vi "MGI CheckValue Directory Calculate.vi"(5 "U32 Slider Ref":refnum<vi>, 7 "CheckValue Type (Checksum)":T1, 8 "error in (no error)":errorcluster, 10 "Directories to Exclude":string[](array[string]), 11 "Path":path) -> (0 "error out":errorcluster, 1 "CheckValue U32[i]":u32[](array[numeric]) format="%.0x", 2 "Relative Path[i]":path[](array[path]), 4 "Aborted?":bool)   [LabVIEW 2020]
doc: "Output an array of all files contained in the specified directory along with a CheckValue for each file. Optional Progress Bar Input is updated if wired, otherwise a progress bar dialog with abort button is shown.\n\nAuthored by Shawn Walpole\nsupport@mooregoodideas.com\nwww.mooregoodideas.com\n\nCopyright (c) 2010, Moore Good Ideas, Inc.\n\nAll rights reserved.\n\nRedistribution and use in source and binary forms, with or without modification, are permitted provided that the following conditions are met:\n\n * Redistributions of source code must retain the above copyright notice, this list of conditions and the following disclaimer.\n * Redistributions in binary form must reproduce the above copyright notice, this list of conditions and the following disclaimer in the documentation and/or other materials provided with the distribution.\n * Neither the name of Moore Good Ideas, Inc. nor the names of its contributors may be used to endorse or promote products derived from this software without specific prior written permission.\n\nTHIS SOFTWARE IS PROVIDED BY THE COPYRIGHT HOLDERS AND CONTRIBUTORS \"AS IS\" AND ANY EXPRESS OR IMPLIED WARRANTIES, INCLUDING, BUT NOT LIMITED TO, THE IMPLIED WARRANTIES OF MERCHANTABILITY AND FITNESS FOR A PARTICULAR PURPOSE ARE DISCLAIMED. IN NO EVENT SHALL THE COPYRIGHT OWNER OR CONTRIBUTORS BE LIABLE FOR ANY DIRECT, INDIRECT, INCIDENTAL, SPECIAL, EXEMPLARY, OR CONSEQUENTIAL DAMAGES (INCLUDING, BUT NOT LIMITED TO, PROCUREMENT OF SUBSTITUTE GOODS OR SERVICES; LOSS OF USE, DATA, OR PROFITS; OR BUSINESS INTERRUPTION) HOWEVER CAUSED AND ON ANY THEORY OF LIABILITY, WHETHER IN CONTRACT, STRICT LIABILITY, OR TORT (INCLUDING NEGLIGENCE OR OTHERWISE) ARISING IN ANY WAY OUT OF THE USE OF THIS SOFTWARE, EVEN IF ADVISED OF THE POSSIBILITY OF SUCH DAMAGE."
uses:
  <userlib>/_MGI/File/Checksum/MGI CheckValue Method Enum.ctl
panel:
  out "Cur File(Rel)":path
  out "ProcessedFiles":i32
  out "TotalFiles":u32
  # "Controls used for local variables"
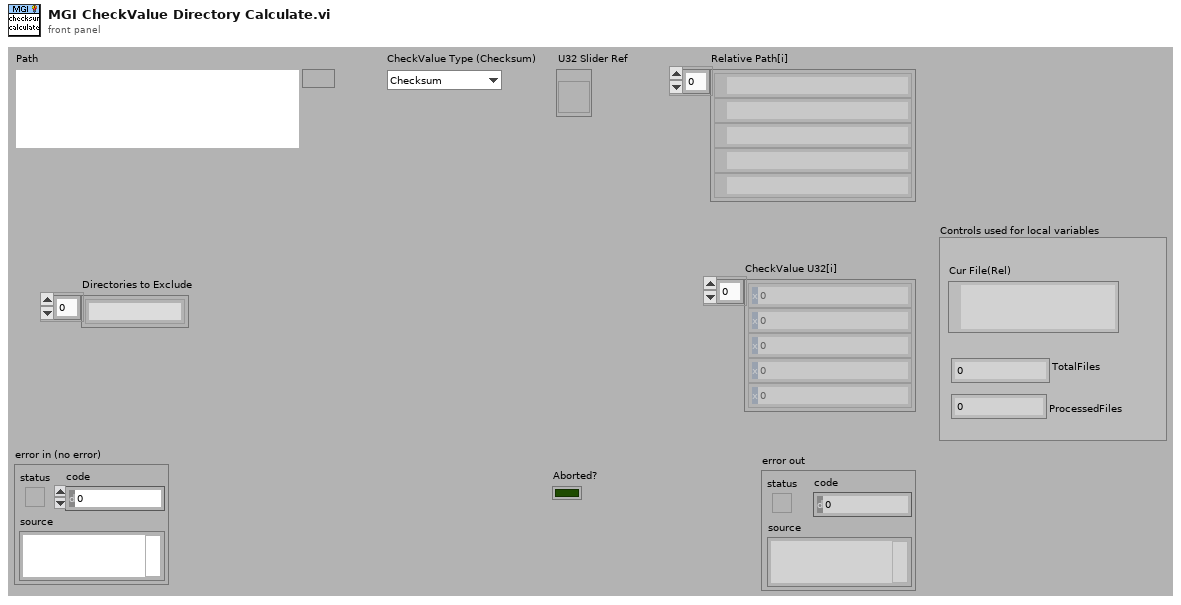
[diagram p1: front panel]
types:
  T1 = typedef "MGI CheckValue Method Enum.ctl" = enum16{"Checksum", "XOr"}
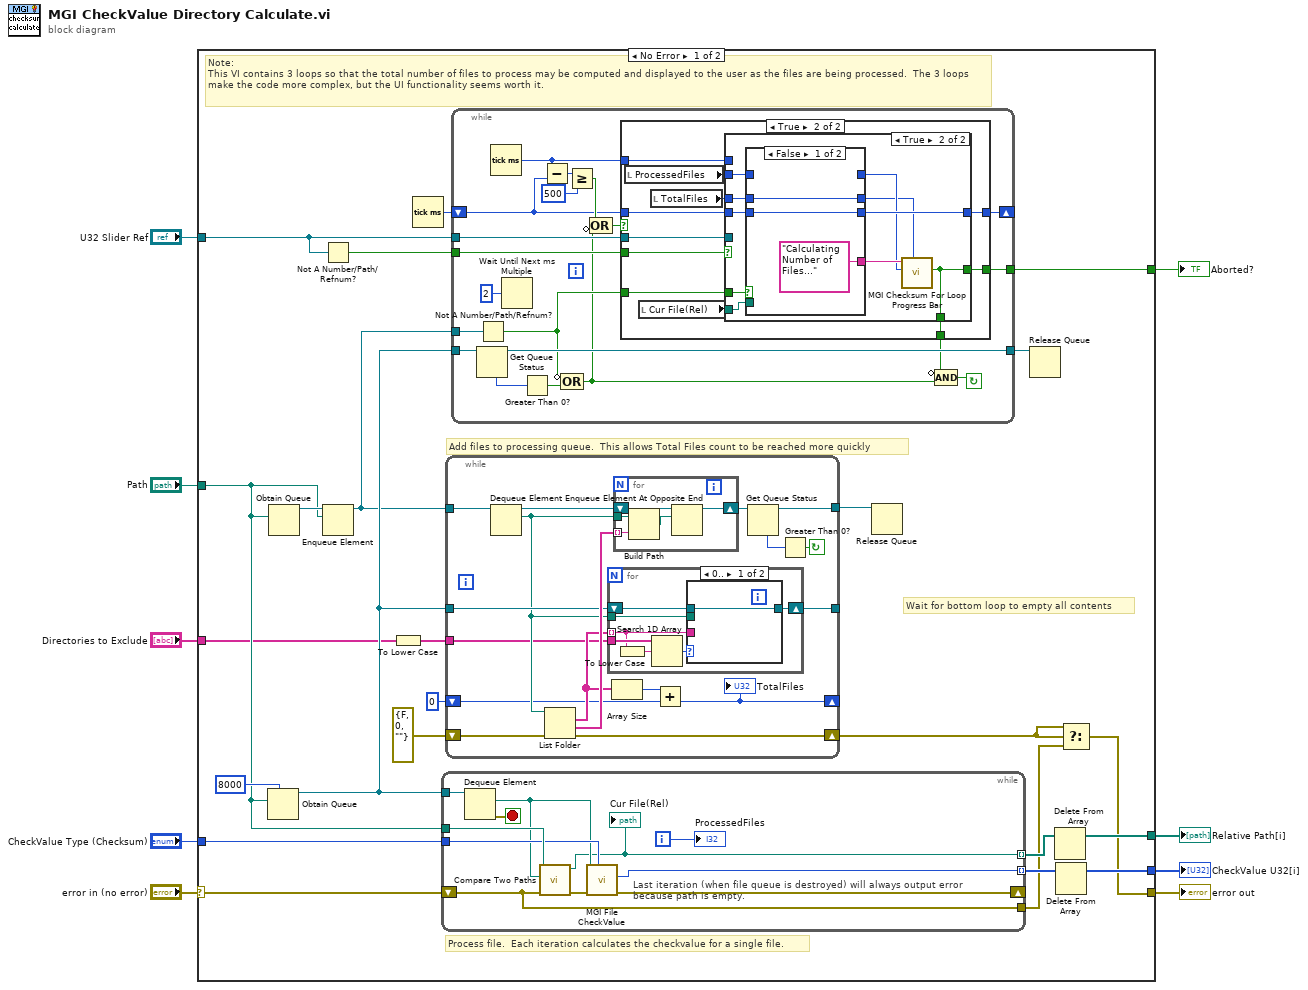
[diagram p0: block diagram]
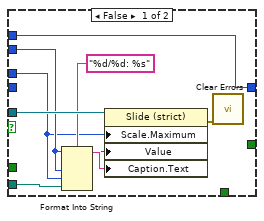
[diagram p3: hidden frame]
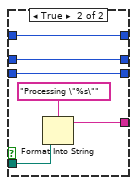
[diagram p4: hidden frame]
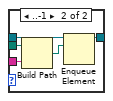
[diagram p5: hidden frame]
diagram:
  n1 = case shown="No Error" "error in (no error)" {
    selector: "error in (no error)" -> [w12 w139]
    tunnel: "Path" -> [w29 _]
    tunnel: "CheckValue Type (Checksum)" -> [w28 _]
    tunnel: [w27 _] -> w7
    tunnel: [w25 _] -> w6
    tunnel: [w21 w139] -> w5
    tunnel: "U32 Slider Ref" -> [w20 _]
    tunnel: [w13 _] -> w2
    tunnel: "Directories to Exclude" -> [w11 _]
    frame No Error {
      # "Note:\nThis VI contains 3 loops so that the total number of files to process may be computed and displayed to the user as the files are being processed.  The 3 loops make the code more complex, but the UI functionality seems worth it."
      # "Process file.  Each iteration calculates the checkvalue for a single file."
      # "Add files to processing queue.  This allows Total Files count to be reached more quickly"
      # "Wait for bottom loop to empty all contents"
      n2 = Obtain Queue(max queue size (-1, unlimited)=8000, element data type=w29) -> (queue out=w19:refnum<queue>)  [unwired: 3 in, 2 out]
      n3 = Obtain Queue(element data type=w29) -> (queue out=w33:refnum<queue>)  [unwired: 4 in, 2 out]
      n4 = Not A Number/Path/Refnum?(number/path/refnum=w20) -> (NaN/Path/Refnum?=w17:bool)
      n5 = Enqueue Element(queue=w33, element=w29) -> (queue out=w18:refnum<queue>)  [unwired: 2 in, 2 out]
      n6 = To Lower Case(string=w11) -> (all lower case string=w10:string[])
      n7 = Tick Count (ms)() -> (millisecond timer value=w16:u32)
      n8 = while {
        shift-right: [w132] -> _
        shift-left: w12 -> [w129]
        tunnel: w19 -> [w138]
        tunnel: w29 -> [w137]
        tunnel: w28 -> [w136]
        tunnel: [w133] -> w24 mode=indexing
        tunnel: [w130] -> w26 mode=indexing
        tunnel: [w129] -> w22
        i -> [w131]
        stop <- w128 stop-if-true
        # "Last iteration (when file queue is destroyed) will always output error because path is empty."
        n9 = Dequeue Element(queue=w138) -> (element=w135:path, error out=w128:errorcluster)  [unwired: 2 in, 2 out]
        n10 = call <vilib>:"Compare Two Paths.vi"("error in (no error)"=w129, "Path 2"=w135, "Path 1"=w137) -> ("error out"=w134:errorcluster, "Relative Path from 1 to 2"=w130:path)  [unwired: 5 in, 2 out]
        "Cur File(Rel)" <- w130
        n11 = call <userlib>:"MGI File CheckValue.vi"("CheckValue Type"=w136, "error in (no error)"=w134, "File"=w135) -> ("error out"=w132:errorcluster, "CheckSum"=w133:u32)  [unwired: 7 in]
        "ProcessedFiles" <- w131
      }
      n12 = while {
        tunnel: w19 -> [w102]
        tunnel: w18 -> [w109]
        shift-right: [w95] -> w23
        shift-left: errorcluster {"status"=FALSE, "code"=0, "source"=""} ("error out") -> [w96]
        tunnel: [w103] -> w15
        shift-right: [w98] -> _
        shift-left: u32 0 -> [w97]
        tunnel: [w94] -> _
        tunnel: w10 -> [w93]
        stop <- w104 continue-if-true
        n13 = Dequeue Element(queue=w109) -> (queue out=w108:refnum<queue>, element=w101:path)  [unwired: 2 in, 2 out]
        n14 = List Folder(path=w101, error in=w96) -> (filenames=w100:string[], folder names=w107:string[], error out=w95:errorcluster)  [unwired: 2 in, 1 out]
        n15 = for {
          tunnel: w100 -> [w111] mode=indexing
          tunnel: w101 -> [w116]
          shift-right: [w114] -> w94
          shift-left: w102 -> [w115]
          tunnel: w93 -> [w112]
          n16 = To Lower Case(string=w111) -> (all lower case string=w110:string)
          n17 = Search 1D Array(1D array=w112, element=w110) -> (index of element=w113:i32)  [unwired: 1 in]
          n18 = case shown="0.." w113 {
            tunnel: w116 -> [_ w122]
            tunnel: w111 -> [_ w121]
            tunnel: w115 -> [w117 w120]
            tunnel: [w117 w118] -> w114
            frame 0.. {
            }
            frame ..-1 {
              n19 = Build Path(base path=w122, name or relative path=w121) -> (appended path=w119:path)
              n20 = Enqueue Element(queue=w120, element=w119) -> (queue out=w118:refnum<queue>)  [unwired: 2 in, 2 out]
            }
          }
        }
        n21 = Array Size(array=w100) -> (size(s)=w99:i32)
        n22 = for {
          tunnel: w107 -> [w126] mode=indexing
          tunnel: w101 -> [w127]
          shift-right: [w123] -> w106
          shift-left: w108 -> [w125]
          n23 = Build Path(base path=w127, name or relative path=w126) -> (appended path=w124:path)
          n24 = Enqueue Element At Opposite End(queue=w125, element=w124) -> (queue out=w123:refnum<queue>)  [unwired: 2 in, 2 out]
        }
        n25 = Add(x=w99, y=w97) -> (x+y=w98:u32)
        "TotalFiles" <- w98
        n26 = Get Queue Status(queue=w106) -> (queue out=w103:refnum<queue>, # elements in queue=w105:i32)  [unwired: 2 in, 6 out]
        n27 = Greater Than 0?(x=w105) -> (x > 0?=w104:bool)
      }
      n28 = while {
        tunnel: w19 -> [w53]
        tunnel: [w50] -> w14
        shift-right: [w49] -> _
        shift-left: w16 -> [w45]
        tunnel: w20 -> [w43]
        tunnel: w18 -> [w41]
        tunnel: w17 -> [w39]
        tunnel: [w34] -> w13
        stop <- w35 continue-if-true
        n29 = Get Queue Status(queue=w53) -> (queue out=w50:refnum<queue>, # elements in queue=w52:i32)  [unwired: 2 in, 6 out]
        n30 = Not A Number/Path/Refnum?(number/path/refnum=w41) -> (NaN/Path/Refnum?=w38:bool)
        n31 = Tick Count (ms)() -> (millisecond timer value=w44:u32)
        n32 = Wait Until Next ms Multiple(millisecond multiple=u32 2) -> ()  [unwired: 1 out]
        n33 = Greater Than 0?(x=w52) -> (x > 0?=w42:bool)
        n34 = Subtract(x=w44, y=w45) -> (x-y=w46:u32)
        n35 = Compound Arithmetic op=OR(invert w38, w42) -> (w37:bool)
        n36 = Greater Or Equal?(x=w46, y=u32 500) -> (x >= y?=w48:bool)
        n37 = Compound Arithmetic op=OR(w48, invert w37) -> (w40:bool)
        n38 = case shown="True" w40 {
          tunnel: [w54 w65] -> w49
          tunnel: w45 -> [w54 w64]
          tunnel: w44 -> [_ w63]
          tunnel: w43 -> [_ w62]
          tunnel: w39 -> [_ w61]
          tunnel: w38 -> [_ w60]
          tunnel: [_ w56] -> w36
          tunnel: [_ w55] -> w34
          frame False {
          }
          frame True {
            n39 = local read "ProcessedFiles"() -> (w59:i32)
            n40 = local read "Cur File(Rel)"() -> (w57:path)
            n41 = local read "TotalFiles"() -> (w58:u32)
            n42 = case shown="True" w61 {
              tunnel: w63 -> [w73 _]
              tunnel: [w73 w81] -> w65
              tunnel: w64 -> [_ w82]
              tunnel: w62 -> [w72 _]
              tunnel: w60 -> [_ w83]
              tunnel: w59 -> [w68 w80]
              tunnel: w58 -> [w67 w79]
              tunnel: w57 -> [w66 w78]
              tunnel: [_ w77] -> w56
              tunnel: [_ w77] -> w55
              frame False {
                n43 = Format Into String(format string="%d/%d: %s", w68, w67, w66) -> (resulting string=w69:string)  [unwired: 2 in, 1 out]
                n44 = property class="Slide (strict)"(reference=w72, "Scale.Maximum"=w67, "Value"=w68, "Caption.Text"=w69) -> (error out=w71:errorcluster)  [unwired: 1 in, 1 out]
                n45 = call <vilib>:"Clear Errors.vi"("error in (no error)"=w71) -> ()  [unwired: 5 in, 2 out]
              }
              frame True {
                n46 = case shown="False" w83 {
                  tunnel: w82 -> [w86 w92]
                  tunnel: [w86 w92] -> w81
                  tunnel: w80 -> [_ w91]
                  tunnel: [_ w91] -> w75
                  tunnel: w79 -> [w84 w90]
                  tunnel: [w84 w90] -> w74
                  tunnel: w78 -> [_ w89]
                  tunnel: ["Calculating Number of Files..." w87] -> w76
                  frame False {
                  }
                  frame True {
                    n47 = Format Into String(format string="Processing \"%s\"", w89) -> (resulting string=w87:string)  [unwired: 2 in, 1 out]
                  }
                }
                n48 = call <userlib>:"MGI Checksum For Loop Progress Bar.vi"("Total Iter"=w74, "Current Iter"=w75, "Message"=w76) -> ("Aborted?"=w77:bool)  [unwired: 7 in, 1 out]
              }
            }
          }
        }
        n49 = Compound Arithmetic op=AND(invert w36, w37) -> (w35:bool)
      }
      n50 = Release Queue(queue=w15) -> ()  [unwired: 2 in, 3 out]
      n51 = Release Queue(queue=w14) -> ()  [unwired: 2 in, 3 out]
      n52 = Delete From Array(array=w26) -> (array with subset deleted=w27:path[])  [unwired: 2 in, 1 out]
      n53 = Delete From Array(array=w24) -> (array with subset deleted=w25:u32[])  [unwired: 2 in, 1 out]
      n54 = Select(t=w23, s=w23, f=w22) -> (s? t:f=w21:errorcluster)
    }
    frame Error {
    }
  }
  "error out" <- w5
  "Relative Path[i]" <- w7
  "CheckValue U32[i]" <- w6
  "Aborted?" <- w2
